vi "BuildMScript.vi"(8 "error in":errorcluster, 10 "string":string, 11 "path":path) -> (0 "error out":errorcluster, 3 "appended path":path)   [LabVIEW 2023]
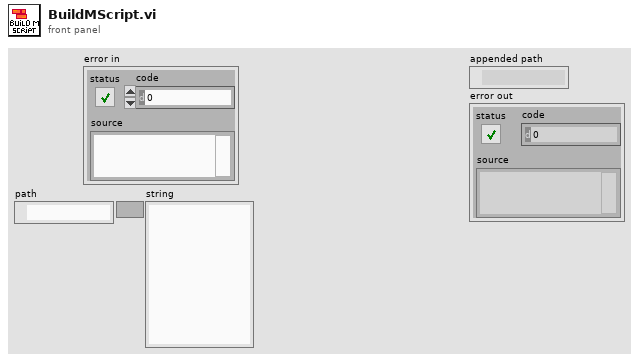
[diagram p1: front panel]
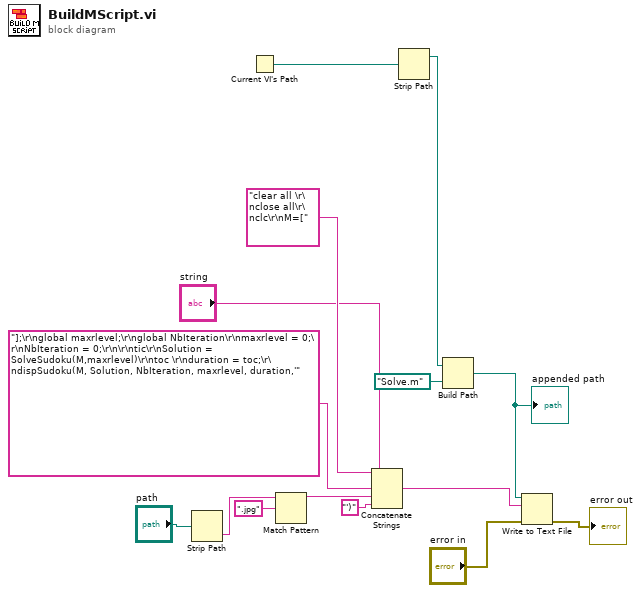
[diagram p0: block diagram]
diagram:
  n1 = Strip Path(path="path") -> (name=w12:string)  [unwired: 1 out]
  n2 = Current VI's Path() -> (path=w7:path)
  n3 = Match Pattern(string=w12, regular expression=".jpg") -> (before substring=w10:string)  [unwired: 1 in, 3 out]
  n4 = Concatenate Strings("clear all \r\nclose all\r\nclc\r\nM=[", "string", "];\r\nglobal maxrlevel;\r\nglobal NbIteration\r\nmaxrlevel = 0;\r\nNbIteration = 0;\r\n\r\ntic\r\nSolution = SolveSudoku(M,maxrlevel)\r\ntoc \r\nduration = toc;\r\ndispSudoku(M, Solution, NbIteration, maxrlevel, duration,'", w10, "')") -> (w6:string)
  n5 = Strip Path(path=w7) -> (stripped path=w8:path)  [unwired: 1 out]
  n6 = Build Path(base path=w8, name or relative path=path "Solve.m") -> (appended path=w5:path)
  "appended path" <- w5
  n7 = Write to Text File(file (use dialog)=w5, text=w6, error in="error in") -> (error out=→"error out":errorcluster)  [unwired: 1 in, 2 out]
